vi "Connection Manager (sound card).vi"(11 "Custom Outputs":string[](array[string])) -> ()   [LabVIEW 2015]
panel:
  in  "Hide unused":bool
  in  "Exit":bool
  in  "Save":bool
  # "Outputs"
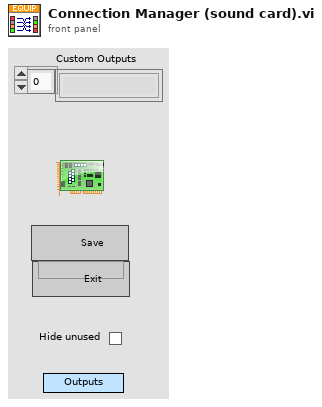
[diagram p1: front panel]
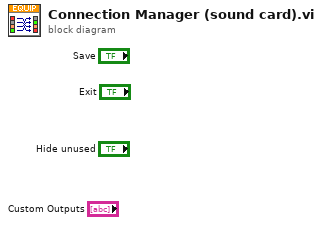
[diagram p0: block diagram]
diagram:
